vi "DHE_DRV_get_mapsize.vi"(11 "error in (no error)":errorcluster) -> (8 "return value":i32, 15 "error out":errorcluster)   [LabVIEW 2016]
doc: "This VI closes the I/O interface with the instrument."
uses:
  c/lib/libarcDHE.so
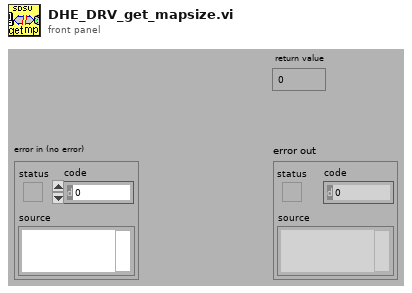
[diagram p1: front panel]
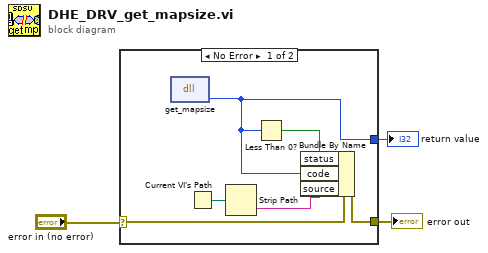
[diagram p0: block diagram]
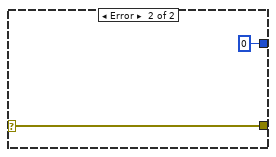
[diagram p2: hidden frame]
diagram:
  n1 = case shown="No Error" "error in (no error)" {
    selector: "error in (no error)" -> [w4 w11]
    tunnel: [w8 0 ("return type")] -> w3
    tunnel: [w5 w11] -> w2
    frame No Error {
      n2 = dll-call lib="home/simager/panview/PAN/Modules/SDSU/private/c/lib/libarcDHE.so" fn="get_mapsize" label="get_maping_size"() -> ("return type"=w8:i32)  [unwired: 3 in, 2 out]
      n3 = Current VI's Path() -> (path=w7:path)
      n4 = Strip Path(path=w7) -> (name=w6:string)  [unwired: 1 out]
      n5 = Less Than 0?(x=w8) -> (x < 0?=w9:bool)
      n6 = Bundle By Name(cluster=w4, "status"=w9, "code"=w8, "source"=w6) -> (w5:errorcluster)
    }
    frame Error {
    }
  }
  "error out" <- w2
  "return value" <- w3
